vi "MessageBase.getOrderedFieldSpecs.vi"(8 "error in (no error)":errorcluster, 11 "MessageBase in":refnum<class "MessageBase.lvclass">) -> (0 "error out":errorcluster, 2 "OrderedFieldSpecs":T1[](array[typedef]), 3 "MessageBase out":refnum<class "MessageBase.lvclass">)   [LabVIEW 2020, in "MessageBase.lvclass"]
uses:
  MessageBase.lvclass
  FieldSpec.ctl
  MessageBase.lvclass/MessageBase.ctl
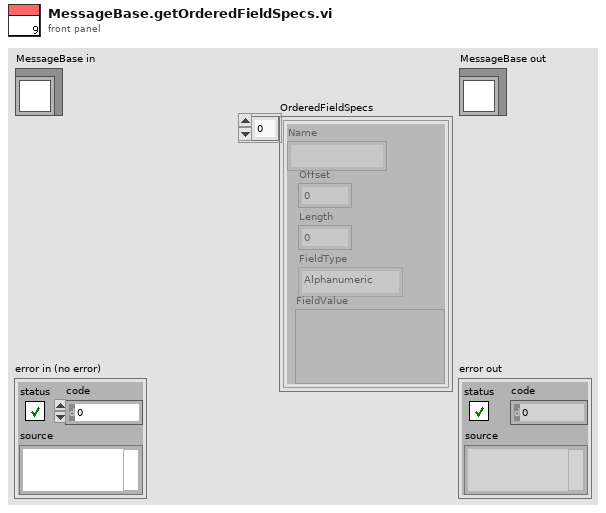
[diagram p1: front panel]
types:
  T1 = typedef "FieldSpec.ctl" = cluster{"Name":string, "Offset":i32, "Length":i32, "FieldType":enum16{"Alphanumeric", "Binary", "BinaryLongPrice", "BinaryShortPrice", "BitField", "PrintableAscii", "Value"}, "FieldValue":variant}
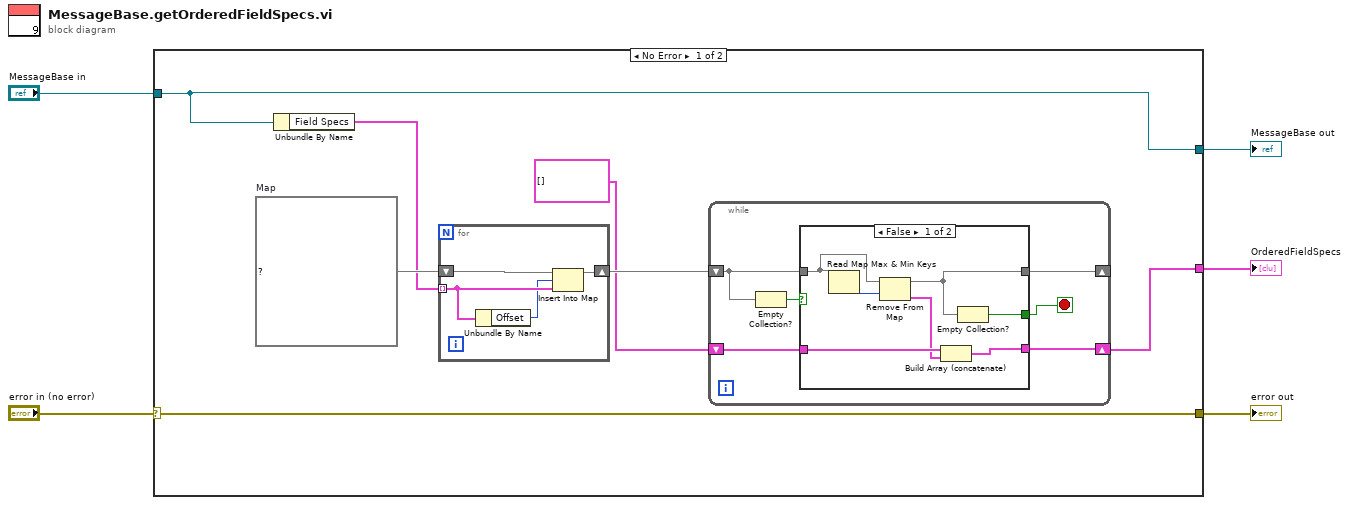
[diagram p0: block diagram]
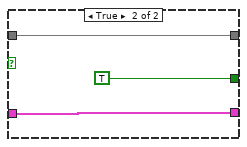
[diagram p2: hidden frame]
diagram:
  n1 = case shown="No Error" "error in (no error)" {
    selector: "error in (no error)" -> [w12 w34]
    tunnel: [w12 w34] -> w4
    tunnel: [w7 w33] -> w2
    tunnel: "MessageBase in" -> [w7 w33]
    tunnel: [w6 _] -> w1
    frame No Error {
      w9 = map{i32, T1} {}  # Map
      n2 = Unbundle By Name(w7) -> ("Field Specs"=w8:T1[])
      n3 = for {
        tunnel: w8 -> [w31] mode=indexing
        shift-right: [w29] -> w11
        shift-left: w9 -> [w32]
        n4 = Unbundle By Name(w31) -> ("Offset"=w30:i32)
        n5 = Insert Into Map(map in=w32, key=w30, value=w31) -> (map out=w29:map{i32, T1})  [unwired: 2 out]
      }
      n6 = while {
        shift-right: [w16] -> _
        shift-left: w11 -> [w15]
        shift-right: [w14] -> w6
        shift-left: T1[] [] -> [w13]
        stop <- w17 stop-if-true
        n7 = Empty Collection?(1:w15) -> (0:w18:bool)
        n8 = case shown="False" w18 {
          tunnel: [w19 TRUE] -> w17
          tunnel: [w20 w27] -> w16
          tunnel: w15 -> [w22 w27]
          tunnel: [w24 w26] -> w14
          tunnel: w13 -> [w25 w26]
          frame False {
            n9 = Read Map Max & Min Keys(11:w22) -> (1:w23:i32)  [unwired: 1 out]
            n10 = Remove From Map(10:w23, 11:w22) -> (1:w21:T1, 3:w20:map{i32, T1})  [unwired: 1 out]
            n11 = Build Array (concatenate)(w25, w21) -> (w24:T1[])
            n12 = Empty Collection?(1:w20) -> (0:w19:bool)
          }
          frame True {
          }
        }
      }
    }
    frame Error {
    }
  }
  "error out" <- w4
  "MessageBase out" <- w2
  "OrderedFieldSpecs" <- w1
